vi "LedTest.vi"() -> ()   [LabVIEW 2018]
panel:
  in  "stop":bool
  in  "Forward Control":bool
  in  "Contact H1":bool=TRUE
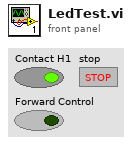
[diagram p1: front panel]
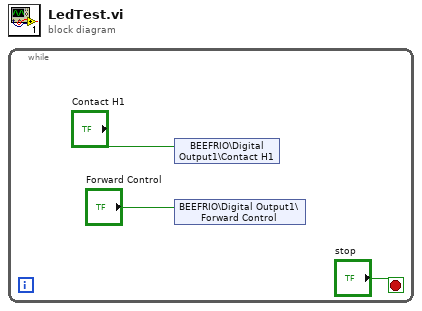
[diagram p0: block diagram]
diagram:
  n1 = while {
    stop <- "stop" stop-if-true
    n2 = shared-variable "BEEFRIO\\Digital Output1\\Contact H1"("Contact H1") -> ()  [unwired: 1 in, 1 out]
    n3 = shared-variable "BEEFRIO\\Digital Output1\\Forward Control"("Forward Control") -> ()  [unwired: 1 in, 1 out]
  }
